vi "Read Serial Number.vi"(6 "error in":errorcluster, 8 "MaxRead":i32, 9 "Channel in":u16) -> (0 "error out":errorcluster, 1 "Messages":T1(array[cluster]), 2 "Pass":bool, 3 "Channel out":u16, 4 "Serial Number":string)   [LabVIEW 2023]
uses:
  4f930f32-d09a-43ef-bca1-8b214b378bd5.vi
  e8470de1-fa2d-4ee3-b50e-96bd89dc731f.vi
  d0f02419-cfb7-4a5e-bc3c-f035efdb0e96.vi
  Communication/PCAN2023/PCAN API.lvlib
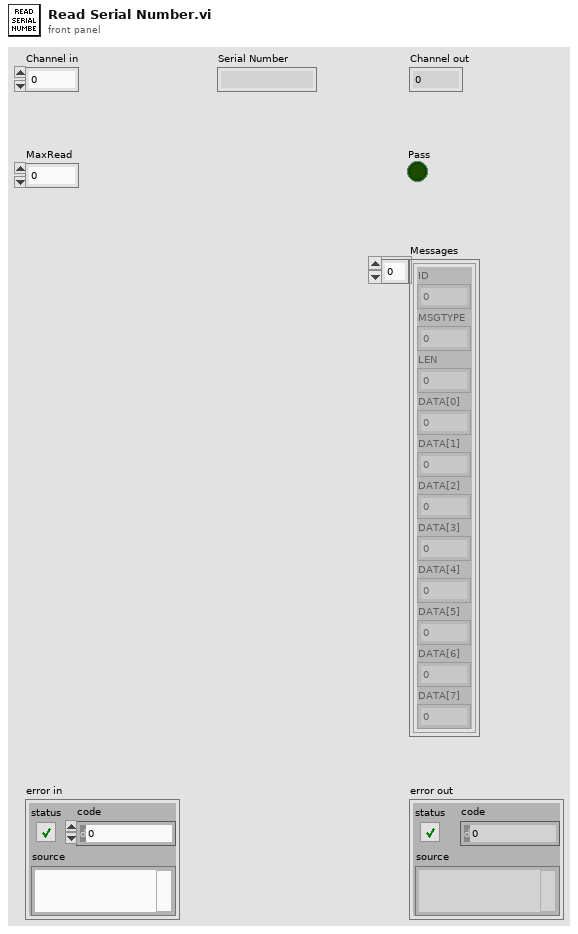
[diagram p1: front panel]
types:
  T1 = cluster{"ID":u32, "MSGTYPE":u8, "LEN":u8, "DATA[0]":u8, "DATA[1]":u8, "DATA[2]":u8, "DATA[3]":u8, "DATA[4]":u8, "DATA[5]":u8, "DATA[6]":u8, "DATA[7]":u8}[]
  T2 = cluster{"ID":u32, "MSGTYPE":u8, "LEN":u8, "DATA[0]":u8, "DATA[1]":u8, "DATA[2]":u8, "DATA[3]":u8, "DATA[4]":u8, "DATA[5]":u8, "DATA[6]":u8, "DATA[7]":u8}
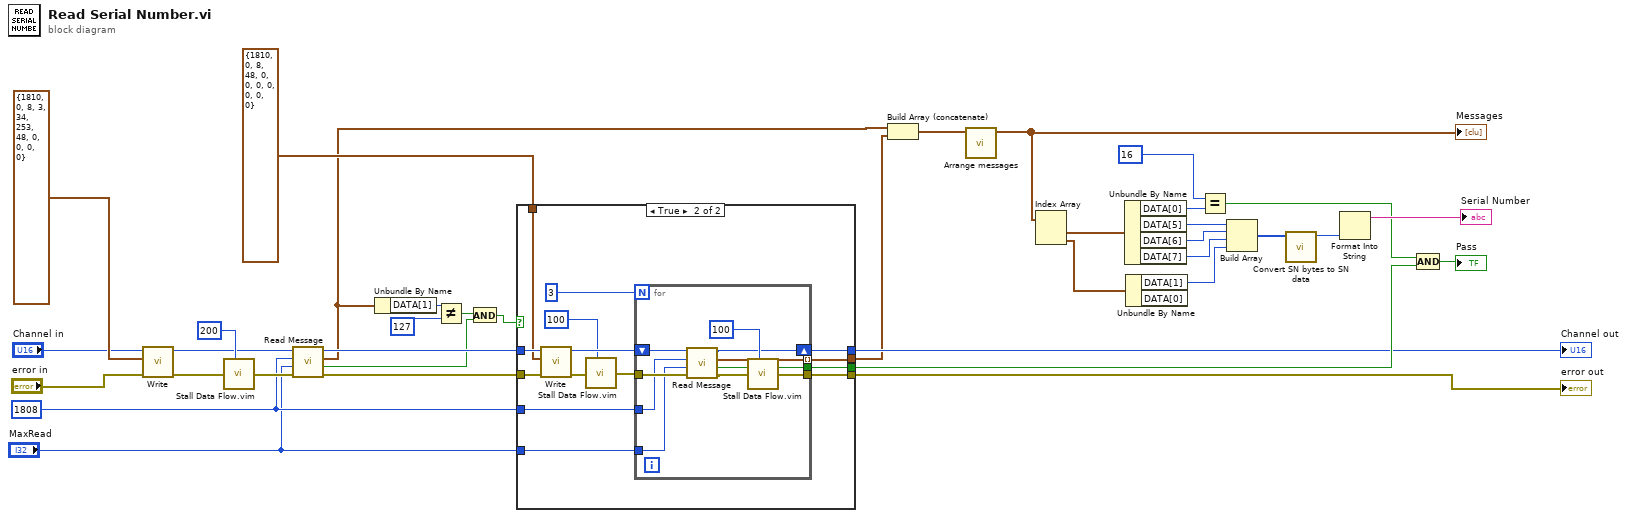
[diagram p0: block diagram]
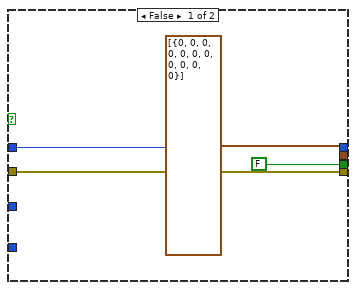
[diagram p2: hidden frame]
diagram:
  (unwired) u32 200 ("milliseconds to wait")
  w9 = u32 1808 ("ID")
  n1 = call "Write.vi"("error in"="error in", "MessageBuffer"=T2 {"ID"=1810, "MSGTYPE"=0, "LEN"=8, "DATA[0]"=3, "DATA[1]"=34, "DATA[2]"=253, "DATA[3]"=48, "DATA[4]"=0, "DATA[5]"=0, "DATA[6]"=0, "DATA[7]"=0}, "Channel"="Channel in") -> ("error out"=w32:errorcluster, "Channel out"=w14:u16)  [unwired: 5 in, 2 out]
  n2 = call "Stall Data Flow.vim"("value in"=w32, "milliseconds to wait"=u32 200) -> ("value out"=w12:errorcluster)  [unwired: 1 out]
  n3 = call "Read Message.vi"("error in"=w12, "MaxRead"="MaxRead", "ID"=w9, "Channel in"=w14) -> ("error out"=w11:errorcluster, "Passed"=w6:bool, "Last Message"=w10:T2, "Channel out"=w13:u16)  [unwired: 3 in, 1 out]
  n4 = Unbundle By Name(w10) -> ("DATA[1]"=w27:u8)
  n5 = Not Equal?(x=w27, y=u8 127) -> (x != y?=w7:bool)
  n6 = And(x=w7, y=w6) -> (x .and. y?=w5:bool)
  n7 = case shown="True" w5 {
    tunnel: w13 -> [w40 w55]
    tunnel: w11 -> [w38 w54]
    tunnel: [w38 w53] -> w31
    tunnel: [FALSE w52] -> w30
    tunnel: [w40 w50] -> w29
    tunnel: T2 {"ID"=1810, "MSGTYPE"=0, "LEN"=8, "DATA[0]"=48, "DATA[1]"=0, "DATA[2]"=0, "DATA[3]"=0, "DATA[4]"=0, "DATA[5]"=0, "DATA[6]"=0, "DATA[7]"=0} ("MessageBuffer") -> [_ w48]
    tunnel: [T1 [{"ID"=0, "MSGTYPE"=0, "LEN"=0, "DATA[0]"=0, "DATA[1]"=0, "DATA[2]"=0, "DATA[3]"=0, "DATA[4]"=0, "DATA[5]"=0, "DATA[6]"=0, "DATA[7]"=0}] w44] -> w15
    tunnel: w9 -> [_ w43]
    tunnel: "MaxRead" -> [_ w42]
    frame False {
    }
    frame True {
      n8 = call "Write.vi"("error in"=w54, "MessageBuffer"=w48, "Channel"=w55) -> ("error out"=w45:errorcluster, "Channel out"=w51:u16)  [unwired: 5 in, 2 out]
      n9 = call "Stall Data Flow.vim"("value in"=w45, "milliseconds to wait"=u32 100) -> ("value out"=w49:errorcluster)  [unwired: 1 out]
      n10 = for {
        N: 3 -> [_]
        tunnel: [w58] -> w52
        shift-right: [w62] -> w50
        shift-left: w51 -> [w63]
        tunnel: w49 -> [w61]
        tunnel: [w65] -> w53
        tunnel: [w59] -> w44 mode=indexing
        tunnel: w43 -> [w57]
        tunnel: w42 -> [w56]
        n11 = call "Read Message.vi"("error in"=w61, "MaxRead"=w56, "ID"=w57, "Channel in"=w63) -> ("error out"=w60:errorcluster, "Passed"=w58:bool, "Last Message"=w59:T2, "Channel out"=w62:u16)  [unwired: 3 in, 1 out]
        n12 = call "Stall Data Flow.vim"("value in"=w60, "milliseconds to wait"=u32 100) -> ("value out"=w65:errorcluster)  [unwired: 1 out]
      }
    }
  }
  "error out" <- w31
  "Channel out" <- w29
  n13 = Build Array (concatenate)(w10, w15) -> (w4:T1)
  n14 = call "Arrange messages.vi"("Array in"=w4) -> ("Array out"=w3:T1)  [unwired: 10 in]
  "Messages" <- w3
  n15 = Index Array(array=w3) -> (element #1=w2:T2, element #2=w1:T2)  [unwired: 2 in]
  n16 = Unbundle By Name(w2) -> ("DATA[0]"=w17:u8, "DATA[5]"=w25:u8, "DATA[6]"=w24:u8, "DATA[7]"=w23:u8)
  n17 = Unbundle By Name(w1) -> ("DATA[1]"=w22:u8)  [unwired: 1 out]
  n18 = Equal?(x=u8 16 ("y"), y=w17) -> (x = y?=w18:bool)
  n19 = Build Array(w25, w24, w23, w22) -> (w21:u8[])
  n20 = call "Convert SN bytes to SN data.vi"("SN Data Bytes"=w21) -> ("SN"=w20:u32)  [unwired: 10 in]
  n21 = Format Into String(w20) -> (resulting string=→"Serial Number":string)  [unwired: 3 in, 1 out]
  n22 = Compound Arithmetic op=AND(w18, w30) -> (→"Pass":bool)
